vi "VScaleInfoNI.vi"(0 "A/D bits":u16, 1 "gain":dbl) -> (6 "vGain scalar":dbl, 7 "vGain (dB)":dbl, 9 "Total Gain (dB)":dbl, 10 "Voltage Scale":T1)   [LabVIEW 2022 SP3]
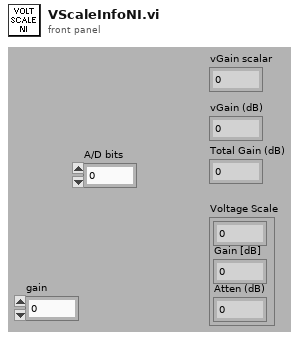
[diagram p1: front panel]
types:
  T1 = cluster{sgl, "Gain [dB]  ":sgl, "Atten (dB)":sgl}
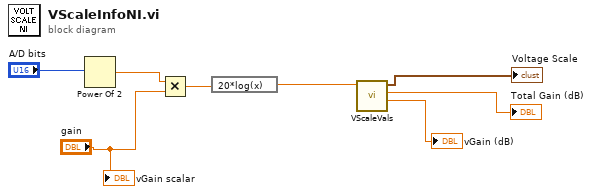
[diagram p0: block diagram]
diagram:
  n1 = Power Of 2(x="A/D bits") -> (2^x=w3:dbl)
  n2 = Multiply(x=w3, y="gain") -> (x*y=w1:dbl)
  n3 = expression code="20*log(x)"(w1) -> (w8:dbl)
  n4 = call "VScaleVals.vi"("Full Scale"=w8) -> ("vGain (dB)"=→"vGain (dB)":dbl, "Total Gain (dB)"=→"Total Gain (dB)":dbl, "Voltage Scale"=→"Voltage Scale":T1)  [unwired: 8 in]
  "vGain scalar" <- "gain"
